vi "set_update_image.vi"(6 "control references":T1, 8 "error in (no error)":errorcluster, 10 "internet version in":string, 11 "update in":T2) -> (0 "error out":errorcluster, 3 "update out":T2)   [LabVIEW 2010, in "HelioUpdateMH100803.lvclass"]
uses:
  HelioUpdateMH100803.lvclass
  main/labview_source/controls/update_picture.ctl
  main/labview_source/type_definitions/clusters/controls_refs.ctl
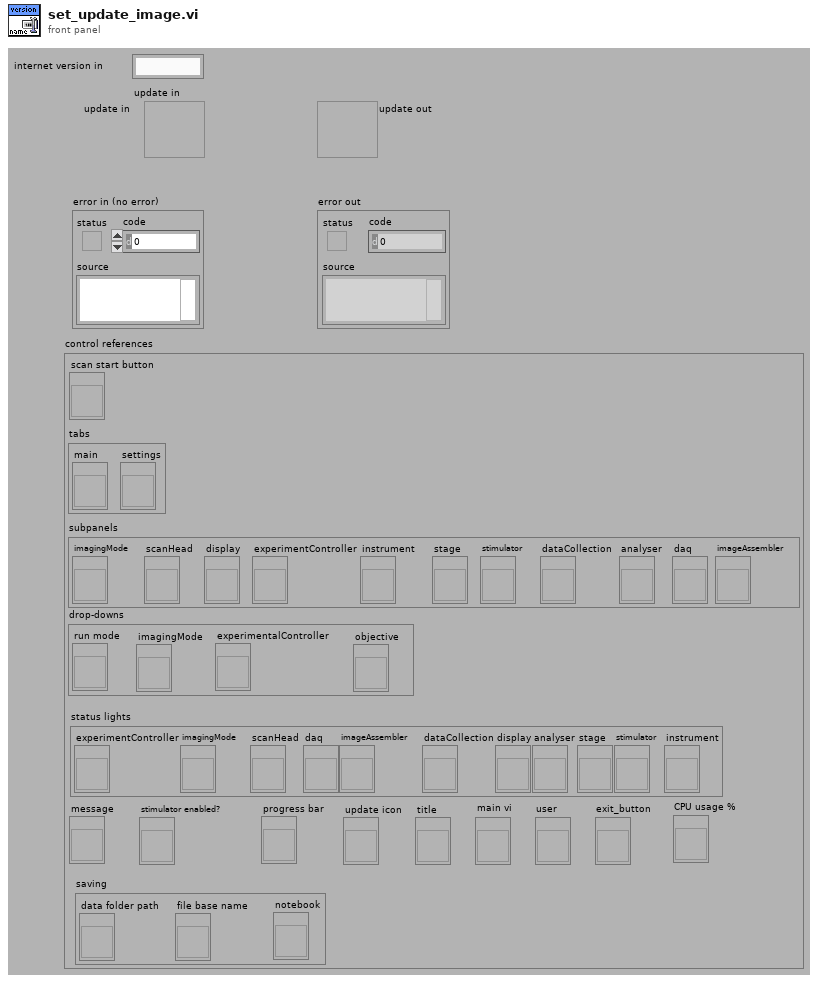
[diagram p1: front panel]
types:
  T1 = typedef "controls_refs.ctl" = cluster{"scan start button":refnum<vi>, "tabs":cluster{"main":refnum<vi>, "settings":refnum<vi>}, "subpanels":cluster{"imagingMode":refnum<vi>, "scanHead":refnum<vi>, "display":refnum<vi>, "experimentController":refnum<vi>, "instrument":refnum<vi>, "stage":refnum<vi>, "stimulator":refnum<vi>, "dataCollection":refnum<vi>, "analyser":refnum<vi>, "daq":refnum<vi>, "imageAssembler":refnum<vi>}, "drop-downs":cluster{"run mode":refnum<vi>, "imagingMode":refnum<vi>, "experimentalController":refnum<vi>, "objective":refnum<vi>}, "status lights":cluster{"experimentController":refnum<vi>, "imagingMode":refnum<vi>, "scanHead":refnum<vi>, "daq":refnum<vi>, "imageAssembler":refnum<vi>, "dataCollection":refnum<vi>, "display":refnum<vi>, "analyser":refnum<vi>, "stage":refnum<vi>, "stimulator":refnum<vi>, "instrument":refnum<vi>}, "message":refnum<vi>, "stimulator enabled?":refnum<vi>, "saving":cluster{"data folder path":refnum<vi>, "file base name":refnum<vi>, "notebook":refnum<vi>}, "progress bar":refnum<vi>, "update icon":refnum<vi>, "title":refnum<vi>, "main vi":refnum<vi>, "user":refnum<vi>, "exit_button":refnum<vi>, "CPU usage %":refnum<vi>}
  T2 = typedef "HelioUpdateMH100803.lvclass/update_picture.ctl" = u16
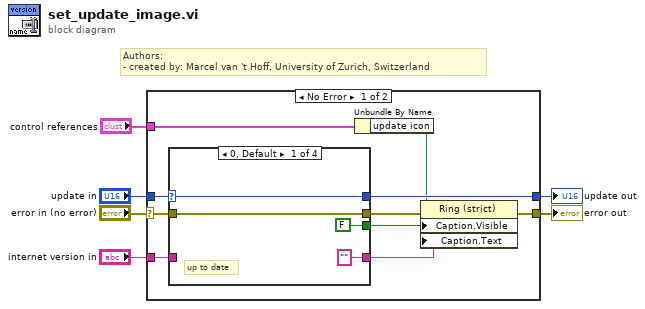
[diagram p0: block diagram]
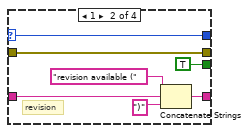
[diagram p2: hidden frame]
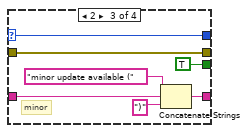
[diagram p3: hidden frame]
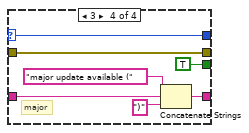
[diagram p4: hidden frame]
diagram:
  # "Authors: \n- created by: Marcel van 't Hoff, University of Zurich, Switzerland"
  n1 = case shown="No Error" "error in (no error)" {
    selector: "error in (no error)" -> [w14 w42]
    tunnel: "update in" -> [w16 _]
    tunnel: "internet version in" -> [w8 _]
    tunnel: [w15 _] -> w3
    tunnel: [w7 w42] -> w2
    tunnel: "control references" -> [w13 _]
    frame No Error {
      n2 = case shown="0, Default" w16 {
        selector: w16 -> [w18 w26 w33 w40]
        tunnel: [FALSE ("Caption.Visible") TRUE ("Caption.Visible") TRUE ("Caption.Visible") TRUE ("Caption.Visible")] -> w10
        tunnel: ["" ("Caption.Text") w21 w28 w35] -> w9
        tunnel: [w18 w26 w33 w40] -> w15
        tunnel: w14 -> [w17 w25 w32 w39]
        tunnel: [w17 w25 w32 w39] -> w11
        tunnel: w8 -> [_ w23 w30 w37]
        frame 0, Default {
          # "up to date"
        }
        frame 1 {
          # "revision"
          n3 = Concatenate Strings("revision available (" ("Caption.Text"), w23, ")" ("string")) -> (w21:string)
        }
        frame 2 {
          # "minor"
          n4 = Concatenate Strings("minor update available (" ("Caption.Text"), w30, ")" ("string")) -> (w28:string)
        }
        frame 3 {
          # "major"
          n5 = Concatenate Strings("major update available (" ("Caption.Text"), w37, ")" ("string")) -> (w35:string)
        }
      }
      n6 = Unbundle By Name(w13) -> ("update icon"=w12:refnum<vi>)
      n7 = property class="Ring (strict)"(reference=w12, error in=w11, "Caption.Visible"=w10, "Caption.Text"=w9) -> (error out=w7:errorcluster)  [unwired: 1 out]
    }
    frame Error {
    }
  }
  "update out" <- w3
  "error out" <- w2
